vi "Get Acknowledgement.vi"(0 "VISA resource name":refnum<visa-resource-name>, 11 "error in (no error)":errorcluster) -> (4 "VISA resource name out":refnum<visa-resource-name>, 15 "error out":errorcluster)   [LabVIEW 2020, in "eec EST 300.lvlib"]
doc: "Reads the response from the instrument, when it is connected in serial mode (This is because the instrument sends the ACK or NACK automatically in this mode of communication)\n\nThis is a Private type VI and meant for getting the acknowledgement alone."
uses:
  <instrlib>/eec EST 300/eec EST 300.lvlib
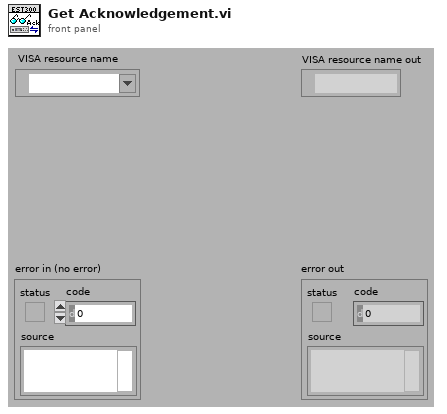
[diagram p1: front panel]
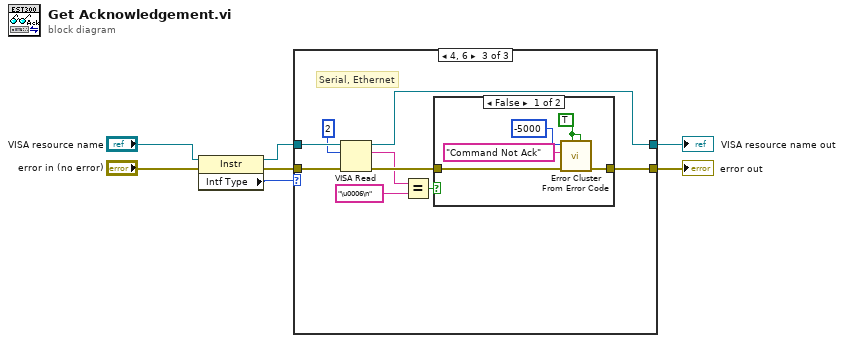
[diagram p0: block diagram]
diagram:
  n1 = property on="Property Node" class="Instr"(reference="VISA resource name", error in="error in (no error)") -> (reference out=w4:refnum<visa-resource-name>, error out=w5:errorcluster, "Intf Type"=w3:u16)
  n2 = case shown="4, 6" w3 {
    tunnel: w4 -> [w9 w11 w19]
    tunnel: [w9 w11 w14] -> w7
    tunnel: w5 -> [w8 w10 w20]
    tunnel: [w8 w10 w16] -> w6
    frame Default {
    }
    frame 1 {
      # "GPIB"
    }
    frame 4, 6 {
      # "Serial, Ethernet"
      n3 = VISA Read(VISA resource name=w19, byte count=u32 2, error in (no error)=w20) -> (VISA resource name out=w14:refnum<visa-resource-name>, read buffer=w12:string, error out=w17:errorcluster)  [unwired: 1 out]
      n4 = Equal?(x=w12, y="\u0006\n") -> (x = y?=w13:bool)
      n5 = case shown="False" w13 {
        tunnel: w17 -> [w25 w26]
        tunnel: [w24 w26] -> w16
        frame False {
          w23 = TRUE ("show call chain? (False)")
          n6 = call <vilib>:"Error Cluster From Error Code.vi"("is warning? (False)"=w23, "show call chain? (False)"=w23, "error in (no error)"=w25, "error message (\"\")"="Command Not Ack" ("error message (\"\")"), "error code (0)"=-5000) -> ("error out"=w24:errorcluster)  [unwired: 4 in]
        }
        frame True {
        }
      }
    }
  }
  "VISA resource name out" <- w7
  "error out" <- w6
